vi "Num of Chan.vi"(8 "error in":errorcluster, 11 "Instrument Handle In":i32) -> (0 "error out":errorcluster, 1 "Ref Channels":i32 caption="Reference Channels", 2 "Input Channels":i32, 3 "Instrument Handle Out":i32, 4 "Calc Channels":i32 caption="Calculation Channels")   [LabVIEW 8.6, in "ZTScopeM.lvlib"]
doc: "Query how many channels the instrument has."
uses:
  ZTScopeM.lvlib
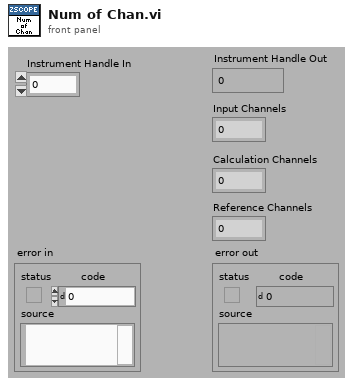
[diagram p1: front panel]
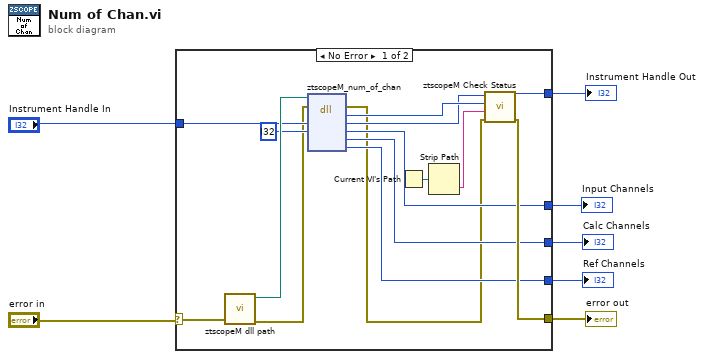
[diagram p0: block diagram]
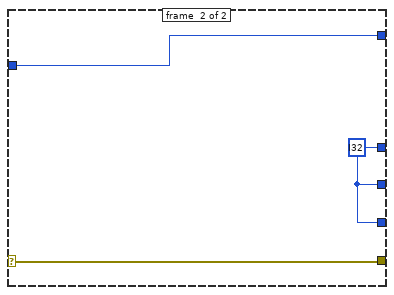
[diagram p2: hidden frame]
diagram:
  n1 = case shown="No Error" "error in" {
    selector: "error in" -> [w16 w25]
    tunnel: [w17 w25] -> w6
    tunnel: [w18 w23] -> w5
    tunnel: "Instrument Handle In" -> [w14 w23]
    tunnel: [w13 w24] -> w3
    tunnel: [w11 w24] -> w2
    tunnel: [w10 w24] -> w1
    frame #0 {
      n2 = call "ztscopeM dll path.vi"("error in (no error)"=w16) -> ("error out"=w9:errorcluster, "<instrument>.dll path"=w15:path)  [unwired: 9 in]
      n3 = dll-call lib="C:/Projects/codedepot/Teradyne/2016-1034 Teradyne ZScope API/Software/ZTScopeM/Public/ztscopeM.dll" fn="ztscopeM_num_of_chan"(path in=w15, error in=w9, "instrumentHandle"=w14, "Input Channels"=i32 ?) -> (error out=w8:errorcluster, "return type"=w22:i32, "instrumentHandle"=w21:i32, "Input Channels"=w13:i32, "Calculation Channels"=w10:i32, "Reference Channels"=w11:i32)  [unwired: 3 in, 1 out]
      n4 = Current VI's Path() -> (path=w20:path)
      n5 = Strip Path(path=w20) -> (name=w19:string)  [unwired: 1 out]
      n6 = call "ztscopeM Check Status.vi"("error in"=w8, "name of VI"=w19, "status (return code)"=w22, "instrument handle in"=w21) -> ("error out"=w17:errorcluster, "instrument handle out"=w18:i32)  [unwired: 2 in]
    }
    frame #1 {
      w24 = i32 ? ("Input Channels")
    }
  }
  "Instrument Handle Out" <- w5
  "error out" <- w6
  "Input Channels" <- w3
  "Ref Channels" <- w2
  "Calc Channels" <- w1
